vi "rotate.vi"(0 "Angle":dbl, 1 "Rate":dbl=-4.0) -> (2 "finished?":bool, 3 "left speed":dbl, 4 "right speed":dbl)   [LabVIEW 2013]
doc: "Rotates the robot for a certain number of degrees at a certain rate."
uses:
  typedefs/Robot Base Width.ctl
  <vilib>/addons/control/pid/pid.llb/PID Control Input Filter (DBL).vi
  <vilib>/addons/control/pid/NI_PID_pid.lvlib
  <vilib>/addons/control/pid/pid.llb/PID (DBL).vi
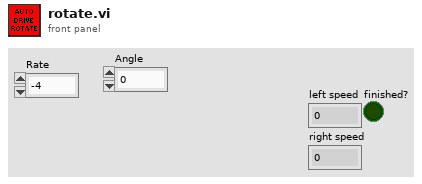
[diagram p1: front panel]
types:
  T1 = typedef "Robot Base Width.ctl" = dbl
  T2 = typedef "subStates.ctl" = enum16{"null", "wait", "driver control", "auto", "manual override", "hold position", "rotate", "pickup", "pass", "load-shoot", "load-pass", "goto shoot", "shoot", "cancel", "end"}
  T3 = typedef "WPI_EncoderDevRef.ctl" = cluster{"DevStatus":errorcluster, "EncoderIndex":T4, "CounterIndex":T5, "DistancePerCount":dbl, "Decoding Type":T6}
  T4 = typedef "FPGA_EncoderIdx.ctl" = enum8{"Enc 0", "Enc 1", "Enc 2", "Enc 3", "Invalid"}
  T5 = typedef "FPGA_CounterCtrSystemIndex.ctl" = enum8{"Ctr 0", "Ctr 1", "Ctr 2", "Ctr 3", "Ctr 4", "Ctr 5", "Ctr 6", "Ctr 7", "Invalid"}
  T6 = typedef "WPI_EncoderType.ctl" = enum16{"1x", "2x", "4x"}
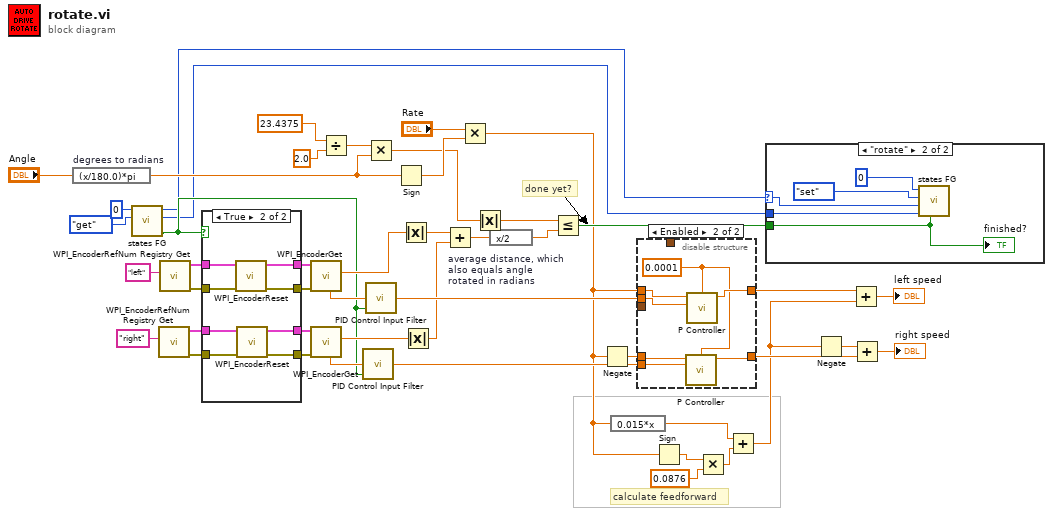
[diagram p0: block diagram]
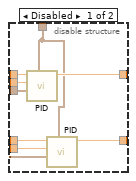
[diagram p2: hidden frame]
diagram:
  # "calculate feedforward"
  # "done yet?"
  n1 = expression code="(x/180.0)*pi" "degrees to radians"("Angle") -> (w5:dbl)
  n2 = call "states FG.vi"("menu (get)"=enum16{"set", "get"}."get", "Loop ID"=0) -> ("first call?"=w20:bool, "state # out"=w3:i32, "subState out"=w2:T2)  [unwired: 6 in, 1 out]
  n3 = call <vilib>:"WPI_EncoderRefNum Registry Get.vi"("refnum name"="right") -> ("error out"=w31:errorcluster, "EncoderDevRef"=w32:T3)  [unwired: 9 in]
  n4 = call <vilib>:"WPI_EncoderRefNum Registry Get.vi"("refnum name"="left") -> ("error out"=w33:errorcluster, "EncoderDevRef"=w34:T3)  [unwired: 9 in]
  n5 = case shown="True" w20 {
    tunnel: w34 -> [w51 w57]
    tunnel: w33 -> [w50 w59]
    tunnel: w32 -> [w49 w54]
    tunnel: w31 -> [w48 w55]
    tunnel: [w50 w58] -> w30
    tunnel: [w51 w56] -> w29
    tunnel: [w49 w53] -> w28
    tunnel: [w48 w52] -> w27
    frame False {
    }
    frame True {
      n6 = call <vilib>:"WPI_EncoderReset.vi"("error in (no error)"=w59, "EncoderDevRef"=w57) -> ("error out"=w58:errorcluster, "EncoderDevRef"=w56:T3)  [unwired: 8 in]
      n7 = call <vilib>:"WPI_EncoderReset.vi"("error in (no error)"=w55, "EncoderDevRef"=w54) -> ("error out"=w52:errorcluster, "EncoderDevRef"=w53:T3)  [unwired: 8 in]
    }
  }
  n8 = call <vilib>:"WPI_EncoderGet.vi"("error in (no error)"=w30, "EncoderDevRef"=w29) -> ("Distance"=w26:dbl, "Rate"=w39:dbl)  [unwired: 4 in, 4 out]
  n9 = call <vilib>:"WPI_EncoderGet.vi"("error in (no error)"=w27, "EncoderDevRef"=w28) -> ("Distance"=w25:dbl, "Rate"=w38:dbl)  [unwired: 4 in, 4 out]
  n10 = Divide(x=T1 23.4375 ("Robot Base Width (in)"), y=2.0) -> (x/y=w46:T1)
  n11 = call-poly <vilib>:"PID Control Input Filter.vi"("reinitialize? (F)"=w20, "input"=w38) -> ("output"=w21:dbl)  [unwired: 3 in]
  n12 = Multiply(x=w46, y=w5) -> (x*y=w17:T1)
  n13 = call-poly <vilib>:"PID Control Input Filter.vi"("reinitialize? (F)"=w20, "input"=w39) -> ("output"=w22:dbl)  [unwired: 3 in]
  n14 = Sign(1:w5) -> (0:w18:dbl)
  n15 = Absolute Value(x=w26) -> (abs(x)=w16:dbl)
  n16 = Absolute Value(x=w25) -> (abs(x)=w15:dbl)
  n17 = Add(x=w16, y=w15) -> (x+y=w37:dbl)
  n18 = Multiply(x="Rate", y=w18) -> (x*y=w11:dbl)
  n19 = Absolute Value(x=w17) -> (abs(x)=w4:T1)
  n20 = expression code="x/2" "average distance, which also equals angle rotated in radians"(w37) -> (w36:dbl)
  n21 = Less Or Equal?(x=w4, y=w36) -> (x <= y?=w35:bool)
  n22 = Negate(x=w11) -> (-x=w14:dbl)
  n23 = expression code="0.015*x"(w11) -> (w9:dbl)
  n24 = disable-structure shown="Enabled" {
    disable-tunnel: [w67 w71] -> w45
    disable-tunnel: [w66 w72] -> w44
    disable-tunnel: _ -> [w65 _]
    disable-tunnel: w22 -> [w64 w73]
    disable-tunnel: w21 -> [w63 w69]
    disable-tunnel: _ -> [w62 _]
    disable-tunnel: w14 -> [w61 w70]
    disable-tunnel: w11 -> [w60 w74]
    frame Disabled {
      n25 = call-poly <vilib>:"PID.vi"("output range"=w65, "PID gains"=w62, "process variable"=w64, "setpoint"=w60) -> ("output"=w66:dbl)  [unwired: 6 in, 1 out]
      n26 = call-poly <vilib>:"PID.vi"("output range"=w65, "PID gains"=w62, "process variable"=w63, "setpoint"=w61) -> ("output"=w67:dbl)  [unwired: 6 in, 1 out]
    }
    frame Enabled {
      w68 = 0.0001 ("proportional gain (Kc)")
      n27 = call "P Controller.vi"("Kp"=w68, "Setpoint"=w70, "Process Variable"=w69) -> ("Output"=w71:dbl)  [unwired: 5 in]
      n28 = call "P Controller.vi"("Kp"=w68, "Setpoint"=w74, "Process Variable"=w73) -> ("Output"=w72:dbl)  [unwired: 5 in]
    }
  }
  n29 = Sign(1:w11) -> (0:w13:dbl)
  n30 = Multiply(x=w13, y=0.0876) -> (x*y=w10:dbl)
  n31 = Add(x=w9, y=w10) -> (x+y=w7:dbl)
  n32 = case shown="\"rotate\"" w2 {
    selector: w2 -> [_ w75]
    tunnel: w35 -> [_ w78]
    tunnel: w3 -> [_ w76]
    frame "null", Default {
    }
    frame "rotate" {
      n33 = call "states FG.vi"("exit in"=w78, "state # in"=w76, "subState in"=w75, "menu (get)"=enum16{"set", "get"}."set", "Loop ID"=0) -> ()  [unwired: 3 in, 4 out]
      "finished?" <- w78
    }
  }
  n34 = Negate(x=w7) -> (-x=w8:dbl)
  n35 = Add(x=w44, y=w7) -> (x+y=→"left speed":dbl)
  n36 = Add(x=w8, y=w45) -> (x+y=→"right speed":dbl)
